vi "Script Menu from Folder_Do.vi"(8 "error in (no error)":errorcluster, 11 "Run Data":T1={"Target Folder"=path "", "Menu Folder"=path "", "Active Folder"=path "", "Config"={"Main"={"Menu Folder"="", "Re-Create Menu Folder?"=FALSE, "Allow mnu replace?"=FALSE, "Relative Link Target"=""}, "File Filter"={"Exclude Prefixes"=[], "Ignore Names"=[], "Include Extensions"=[], "Exclude Postfixes"=[]}, "Folder Filter"={"Exclude Prefixes"=[], "Ignore Names"=[]}, "File Name Edit"={"Pre Split String"="", "Post Split String"="", "Deletion Strings"=[]}, "Folder Name Edit"={"Pre Split String"="", "Post Split String"="", "Deletion Strings"=[]}, "Folder Icon Map"={}, "Default Palette Data"={"Display Name Override"="", "View Format"=2, "Palette Width"=0, "Help Tag"="", "Help File Path"=path "", "Palette Description"=""}, "Default File Data"={"Display Name Override"="", "Place VI Contents?"=FALSE}, "Palette Override map"={}, "File Override map"={}}} {"Config"."Default Palette Data"."View Format" items=["Icons", "Text", "Icons and Text"]}) -> (0 "error out":errorcluster, 2 "All mnu files":path[](array[path]), 3 "Created palette path":path)   [LabVIEW 2019, in "AutoMenuCreator.lvlib"]
uses:
  AutoMenuCreator.lvlib
  Ctl/Ctl_Run Data.ctl
  Ctl/Ctl_Config.ctl
  Ctl/Ctl_Config_Main.ctl
  Ctl/Ctl_Config_File Filter.ctl
  Ctl/Ctl_Config_Folder Filter.ctl
  Ctl/Ctl_Config_Name Edit.ctl
  Ctl/Ctl_Config_Folder Icon Map.ctl
  Ctl/Ctl_Config_Palette Data.ctl
  <vilib>/Palette API/Palette Menu/Public Type Define/View Format.ctl
  Ctl/Ctl_Config_File Data.ctl
  1130bf43-b3aa-4d1e-9766-f88ded913ec6.vi
  <vilib>/Palette API/Palette Menu/Palette Menu.lvlib
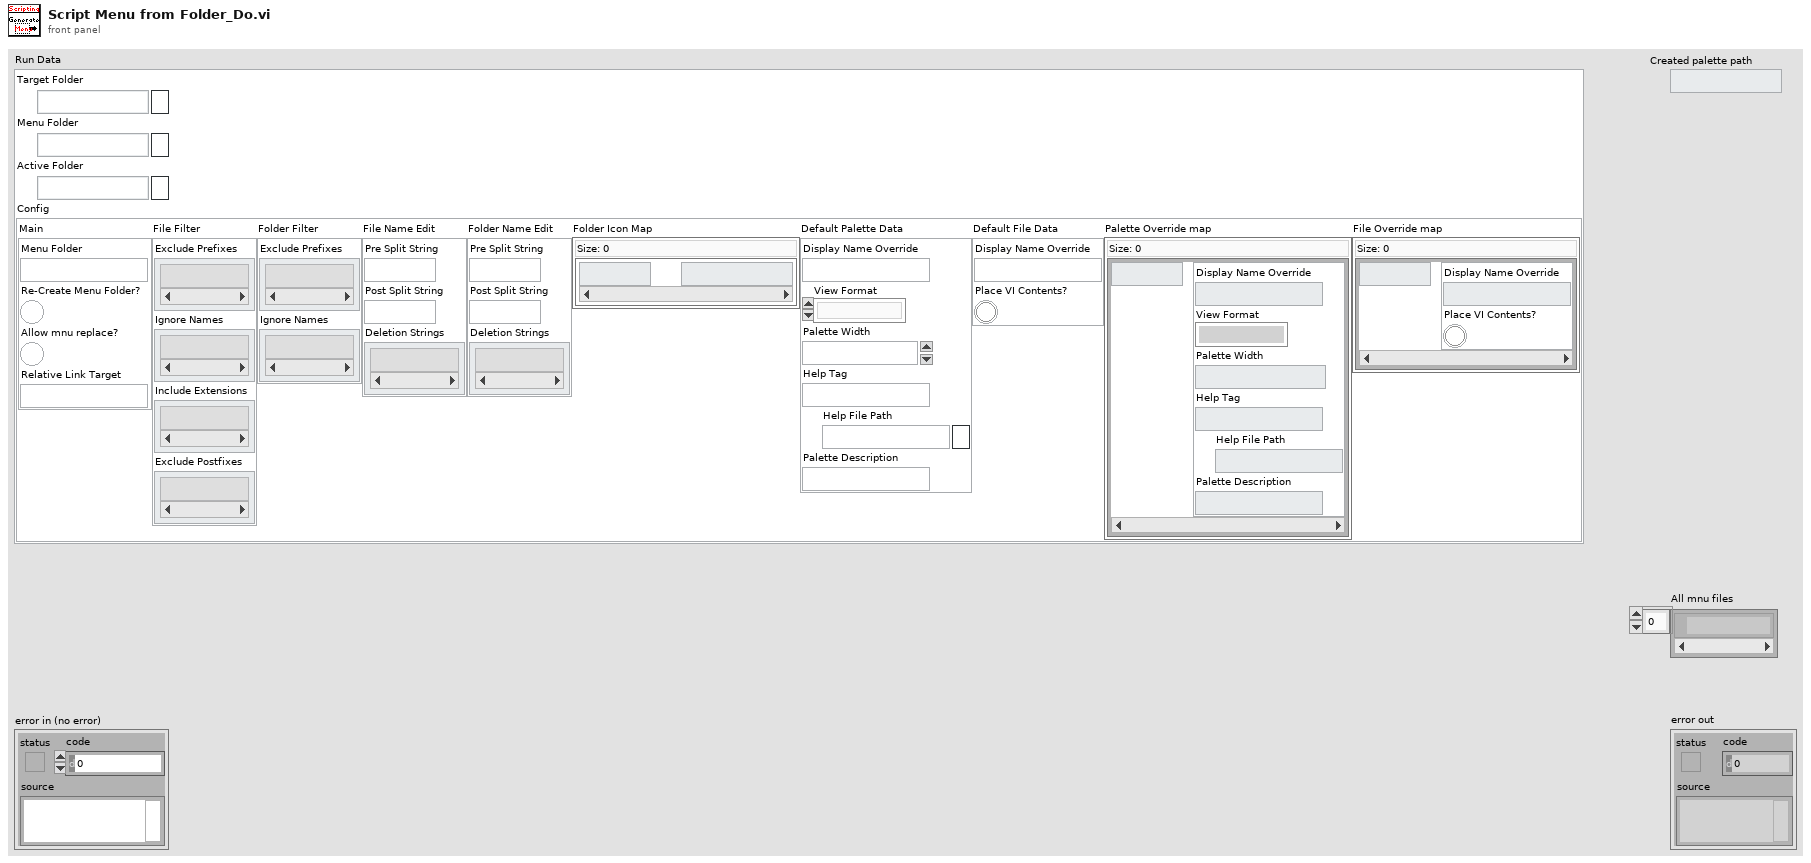
[diagram p1: front panel]
types:
  T1 = typedef "AutoMenuCreator.lvlib/Ctl_Run Data.ctl" = cluster{"Target Folder":path, "Menu Folder":path, "Active Folder":path, "Config":T2}
  T2 = typedef "AutoMenuCreator.lvlib/Ctl_Config.ctl" = cluster{"Main":T3, "File Filter":T4, "Folder Filter":T5, "File Name Edit":T6, "Folder Name Edit":T6, "Folder Icon Map":T7, "Default Palette Data":T8, "Default File Data":T10, "Palette Override map":map{string, T8}, "File Override map":map{string, T10}}
  T3 = typedef "AutoMenuCreator.lvlib/Ctl_Config_Main.ctl" = cluster{"Menu Folder":string, "Re-Create Menu Folder?":bool, "Allow mnu replace?":bool, "Relative Link Target":string}
  T4 = typedef "AutoMenuCreator.lvlib/Ctl_Config_File Filter.ctl" = cluster{"Exclude Prefixes":string[], "Ignore Names":string[], "Include Extensions":string[], "Exclude Postfixes":string[]}
  T5 = typedef "AutoMenuCreator.lvlib/Ctl_Config_Folder Filter.ctl" = cluster{"Exclude Prefixes":string[], "Ignore Names":string[]}
  T6 = typedef "AutoMenuCreator.lvlib/Ctl_Config_Name Edit.ctl" = cluster{"Pre Split String":string, "Post Split String":string, "Deletion Strings":string[]}
  T7 = typedef "AutoMenuCreator.lvlib/Ctl_Config_Folder Icon Map.ctl" = map{string, path}
  T8 = typedef "AutoMenuCreator.lvlib/Ctl_Config_Palette Data.ctl" = cluster{"Display Name Override":string, "View Format":T9, "Palette Width":i16, "Help Tag":string, "Help File Path":path, "Palette Description":string}
  T9 = typedef "Palette Menu.lvlib/View Format.ctl" = u16
  T10 = typedef "AutoMenuCreator.lvlib/Ctl_Config_File Data.ctl" = cluster{"Display Name Override":string, "Place VI Contents?":bool}
  T11 = typedef "Palette Menu.lvlib/Item.ctl" = cluster{"item path":path, "library path":path, "use default lvlib palette":bool, "short name":string, "place VI contents":bool, "hide synchronized item":bool, "reserve spot for synch item":bool, "configure when placing VI contents":bool}
  T12 = typedef "Palette Menu.lvlib/Palette Data.ctl" = cluster{"display name":string, "view format":T9, "palette width":i16, "items":T13, "256 color icon":picture, "B&W color icon":picture, "help information":T14, "palette description":string, "synchronize information":T15}
  T13 = typedef "Palette Menu.lvlib/Items.ctl" = T11[]
  T14 = typedef "Palette Menu.lvlib/Help Info.ctl" = cluster{"help tag":string, "help file path ":path}
  T15 = typedef "Palette Menu.lvlib/Synchronize Info.ctl" = cluster{"synchronize with directory":bool, "synchronize directory path":path}
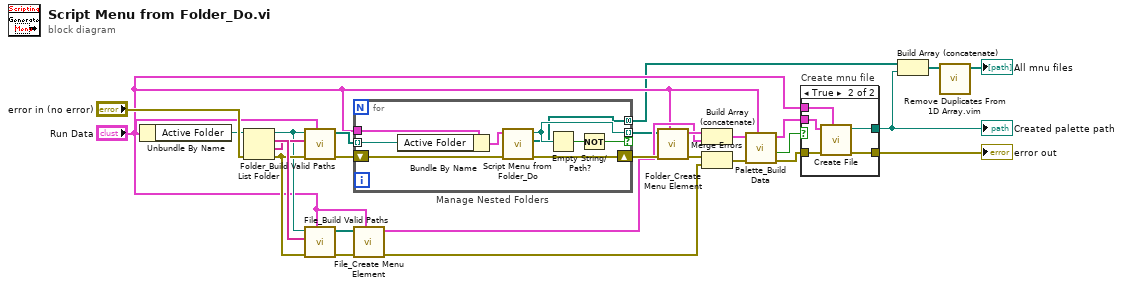
[diagram p0: block diagram]
diagram:
  n1 = Unbundle By Name("Run Data") -> ("Active Folder"=w13:path)
  n2 = List Folder(path=w13, error in="error in (no error)") -> (path out=w14:path, filenames=w27:string[], folder names=w26:string[], error out=w16:errorcluster)  [unwired: 2 in]
  n3 = call "Folder_Build Valid Paths.vi"("Run Data"="Run Data", "error in (no error)"=w16, "Folder names"=w26, "Active Path"=w14) -> ("error out"=w15:errorcluster, "Valid sub-paths"=w24:path[])  [unwired: 6 in]
  n4 = call "File_Build Valid Paths.vi"("Run Data"="Run Data", "error in (no error)"=w16, "File names"=w27, "Active Path"=w14) -> ("error out"=w20:errorcluster, "Valid File Paths"=w25:path[])  [unwired: 6 in]
  n5 = for "Manage Nested Folders" {
    tunnel: w24 -> [w30] mode=indexing
    tunnel: [w35] -> w5 mode=indexing if=w34
    shift-right: [w32] -> w19
    shift-left: w15 -> [w33]
    tunnel: "Run Data" -> [w31]
    tunnel: [w28] -> w1 mode=concatenating
    n6 = Bundle By Name(cluster=w31, "Active Folder"=w30) -> (w29:T1)
    n7 = call "Script Menu from Folder_Do.vi"("error in (no error)"=w33, "Run Data"=w29) -> ("error out"=w32:errorcluster, "All mnu files"=w28:path[], "Created palette path"=w35:path)  [unwired: 7 in]
    n8 = Empty String/Path?(string/path=w35) -> (empty?=w36:bool)
    n9 = Not(x=w36) -> (.not. x?=w34:bool)
  }
  n10 = call "File_Create Menu Element.vi"("Run Data"="Run Data", "error in (no error)"=w20, "Valid File Paths"=w25) -> ("error out"=w17:errorcluster, "Array"=w7:T11[])  [unwired: 7 in]
  n11 = call "Folder_Create Menu Element.vi"("Run Data"="Run Data", "error in (no error)"=w19, "Array in"=w5) -> ("error out"=w18:errorcluster, "Folder Elements out"=w22:T11[])  [unwired: 7 in]
  n12 = Build Array (concatenate)(w22, w7) -> (w8:T11[])
  n13 = Merge Errors(w18, w17) -> (w9:errorcluster)
  n14 = call "Palette_Build Data.vi"("Run Data"="Run Data", "error in (no error)"=w9, "Element Array"=w8) -> ("error out"=w12:errorcluster, "Valid?"=w10:bool, "palette data"=w11:T12)  [unwired: 6 in]
  n15 = case "Create mnu file" shown="True" w10 {
    tunnel: w11 -> [_ w42]
    tunnel: [w37 w41] -> w23
    tunnel: [_ w39] -> w4
    tunnel: w12 -> [w37 w40]
    tunnel: "Run Data" -> [_ w38]
    frame False {
    }
    frame True {
      n16 = call "Create File.vi"("Run Data"=w38, "error in (no error)"=w40, "palette data"=w42) -> ("error out"=w41:errorcluster, "deleted path"=w39:path)  [unwired: 7 in]
    }
  }
  "error out" <- w23
  "Created palette path" <- w4
  n17 = Build Array (concatenate)(w1, w4) -> (w3:path[])
  n18 = call "Remove Duplicates From 1D Array.vim"("array"=w3) -> ("array with duplicates removed"=→"All mnu files":path[])  [unwired: 10 in]
